vi "DequeueMessage.vi"(8 "error in (no error)":errorcluster, 11 "Message Queue In":refnum<queue>) -> (0 "error out":errorcluster, 1 "Data":variant, 2 "Command":string, 3 "Message Queue Out":refnum<queue>)   [LabVIEW 2013, in "Message Queue.lvlib"]
uses:
  Message Queue.lvlib
  ctl_MessageQueue.ctl
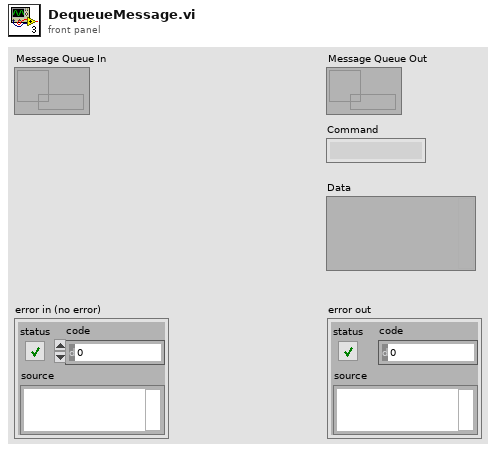
[diagram p1: front panel]
types:
  T1 = typedef "Message Queue.lvlib/ctl_MessageQueue.ctl" = cluster{"Command":string, "Data":variant}
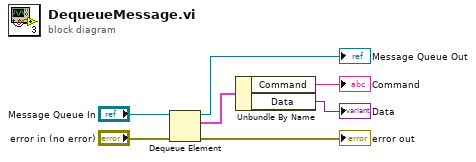
[diagram p0: block diagram]
diagram:
  n1 = Dequeue Element(queue="Message Queue In", error in (no error)="error in (no error)") -> (queue out=→"Message Queue Out":refnum<queue>, element=w6:T1, error out=→"error out":errorcluster)  [unwired: 1 in, 1 out]
  n2 = Unbundle By Name(w6) -> ("Command"=→"Command":string, "Data"=→"Data":variant)
